vi "Loop_ACT_Drive.vi"() -> ()   [LabVIEW 2017]
uses:
  TypeDef/CLUSTER_Drive_HW_SRX_Status.ctl
  TypeDef/CLUSTER_4296_SRX_Status.ctl
  TypeDef/CLUSTER_SRX_Status Data.ctl
  TypeDef/CLUSTER_SRX_Encoder Data.ctl
  TypeDef/CLUSTER_SRX_PWM Data.ctl
  TypeDef/CLUSTER_SRX_Analog Data.ctl
  TypeDef/CLUSTER_SRX_Limit Switch Data.ctl
  TypeDef/CLUSTER_SRX_Profile Data.ctl
  TypeDef/ENUM_Drive_ACT Loop_Mode.ctl
  TypeDef/CLUSTER_Left and Right.ctl
  Globals/Global_STOP.vi
  Global_SM Write_Data Out.vi
  Global_WC_Drive_Zero_Encoders.vi
  Public/Documents/Cross The Road Electronics/Phoenix-LabVIEW/Motor Controller/Get/CTRE_Phoenix_MotorController_GetSelectedSensorData.vi
  Global_WC_Drive_Encoder_Values.vi
  Global_ACT Write_Data Out.vi
panel:
  in  "Zero Encoder":bool
  in  "D":dbl
  in  "I":dbl
  in  "P":dbl
  out "Right Data":dbl
  out "Left Data":dbl
  out "Cycle Time (S)":dbl format="%.3g"
  in  "Target Time(ms)":u32=50
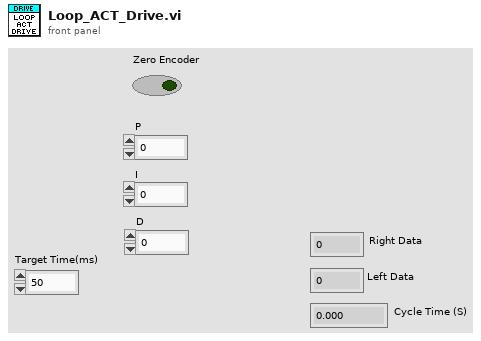
[diagram p1: front panel]
types:
  T1 = typedef "CLUSTER_Left and Right.ctl" = cluster{"Left":dbl, "Right":dbl}
  T2 = typedef "ENUM_Drive_ACT Loop_Mode.ctl" = enum16{"Stop", "Position", "VBus", "Profile"}
  T3 = typedef "CLUSTER_Drive_HW_SRX_Status.ctl" = cluster{"Rear Left":T4, "Rear Right":T4, "Front Left":T4, "Front Right":T4}
  T4 = typedef "CLUSTER_4296_SRX_Status.ctl" = cluster{"Status":T5, "Encoder":T6, "PWM ":T7, "Analog":T8, "Limit Switches":T9, "Profile":T10}
  T5 = typedef "CLUSTER_SRX_Status Data.ctl" = cluster{"Module Enabled":bool, "Current Profile Slot Select":dbl, "Brake is Enabled":bool, "Applied Throttle":dbl, "Current":dbl, "Battery Voltage":dbl, "Sticky Fault - Under Voltage":bool, "Temperature (C)":dbl, "Sticky Fault - Over Temp":bool, "CAN Error":errorcluster, "Control 5 Is Supported":bool}
  T6 = typedef "CLUSTER_SRX_Encoder Data.ctl" = cluster{"Closed Loop Error":dbl, "Sensor Position":dbl, "Sensor Velocity":dbl, "Encoder Position":dbl, "Encoder Velocity":dbl, "Encoder Index Count":dbl, "Encoder A Pin State":bool, "Encoder B Pin State":bool, "Encoder Index Pin State":bool, "Pos Div 8":bool, "Vel Div 4":bool}
  T7 = typedef "CLUSTER_SRX_PWM Data.ctl" = cluster{"Closed Loop Error":dbl, "Pulse Width Position":i32, "Pulse Width Velocity":i32, "Pulse Width Rise To Rise (us)":i32, "Pulse Width Rise To Fall (us)":i32}
  T8 = typedef "CLUSTER_SRX_Analog Data.ctl" = cluster{"Closed Loop Error":dbl, "Analog In":dbl, "Analog In Velocity":dbl}
  T9 = typedef "CLUSTER_SRX_Limit Switch Data.ctl" = cluster{"Forward Limit Switch Closed":bool, "Reverse Limit Switch Closed":bool, "Sticky Fault - Forward Limit":bool, "Sticky Fault - Reverse Limit":bool, "Sticky Fault - Forward Soft Limit":bool, "Sticky Fault - Reverse Soft Limit":bool}
  T10 = typedef "CLUSTER_SRX_Profile Data.ctl" = cluster{"Mot Prof Active Is Under Run":bool, "Mot Prof Active Has Under Run":bool, "Mot Prof Active Is Last":bool, "Mot Prof Active Velocity Only":bool, "Mot Prof Active Is Valid":bool, "Mot Prof Buffer Is Full":bool, "Mot Prof Active Profile Slot Select":i32, "Mot Prof NextID":i32, "Mot Prof Count":i32, "Mot Prof Active Velocity":dbl, "Mot Prof Active Position":dbl, "Mot Prof Output Enable":i32}
  T11 = typedef "WPI_RobotDriveDevRef.ctl" = cluster{"DevStatus":errorcluster, "Motors[]":T12[], "Square Inputs":bool, "Max Output":dbl}
  T12 = typedef "WPI_MotorControlDeviceRef.ctl" = cluster{"DeviceStatus":errorcluster, "Type":T13, "PWM":cluster{"PWM Channel":T14, "DeadBand":T15}, "CAN":cluster{"Device Number":u8, "SetOutput VI Ref":variant, "GetOutput VI Ref":variant, "Enable VI Ref":variant, "Disable VI Ref":variant, "Data":variant}, "Invert":bool, "DIO PWM":cluster{"PWM \"Enable\" Channel":T14, "DIOChannel":T16, "PWM Rate":dbl}}
  T13 = typedef "WPI_MotorControlType.ctl" = enum16{"PWM", "CAN", "DIO PWM"}
  T14 = typedef "FPGA_DIOPWMChannel.ctl" = enum8{"PWM 0", "PWM 1", "PWM 2", "PWM 3", "PWM 4", "PWM 5", "PWM 6", "PWM 7", "PWM 8", "PWM 9", "PWM MXP 0", "PWM MXP 1", "PWM MXP 2", "PWM MXP 3", "PWM MXP 4", "PWM MXP 5", "PWM MXP 6", "PWM MXP 7", "PWM MXP 8", "PWM MXP 9", "Invalid"}
  T15 = typedef "WPI_PWMDeadband.ctl" = cluster{"Name":string, "maxPositivePwm":i32, "minPositivePwm":i32, "centerPwm":i32, "maxNegativePwm":i32, "minNegativePwm":i32, "angularRange":u16}
  T16 = typedef "FPGA_DIOChannel.ctl" = enum8{"DIO 0", "DIO 1", "DIO 2", "DIO 3", "DIO 4", "DIO 5", "DIO 6", "DIO 7", "DIO 8", "DIO 9", "DIO MXP 0", "DIO MXP 1", "DIO MXP 2", "DIO MXP 3", "DIO MXP 4", "DIO MXP 5", "DIO MXP 6", "DIO MXP 7", "DIO MXP 8", "DIO MXP 9", "DIO MXP 10", "DIO MXP 11", "DIO MXP 12", "DIO MXP 13", "DIO MXP 14", "DIO MXP 15", "SPI Port CS1", "SPI Port CS2", "SPI Port CS3", "SPI Port MISO", "SPI Port MOSI", "Invalid"}
  T17 = cluster{"RobotDriveDevRef":T11, "Target Time(ms)":u32, "Current Time":timestamp, "Previous Time":timestamp, "Cycle Time (S)":dbl, "SRX_Status":T3, "Mode":T2, "VBus":T1, "Cruise RPM":dbl, "MAX Velocity\n":dbl, "Encoder Target Position":i32, "Zero Encoder":bool}
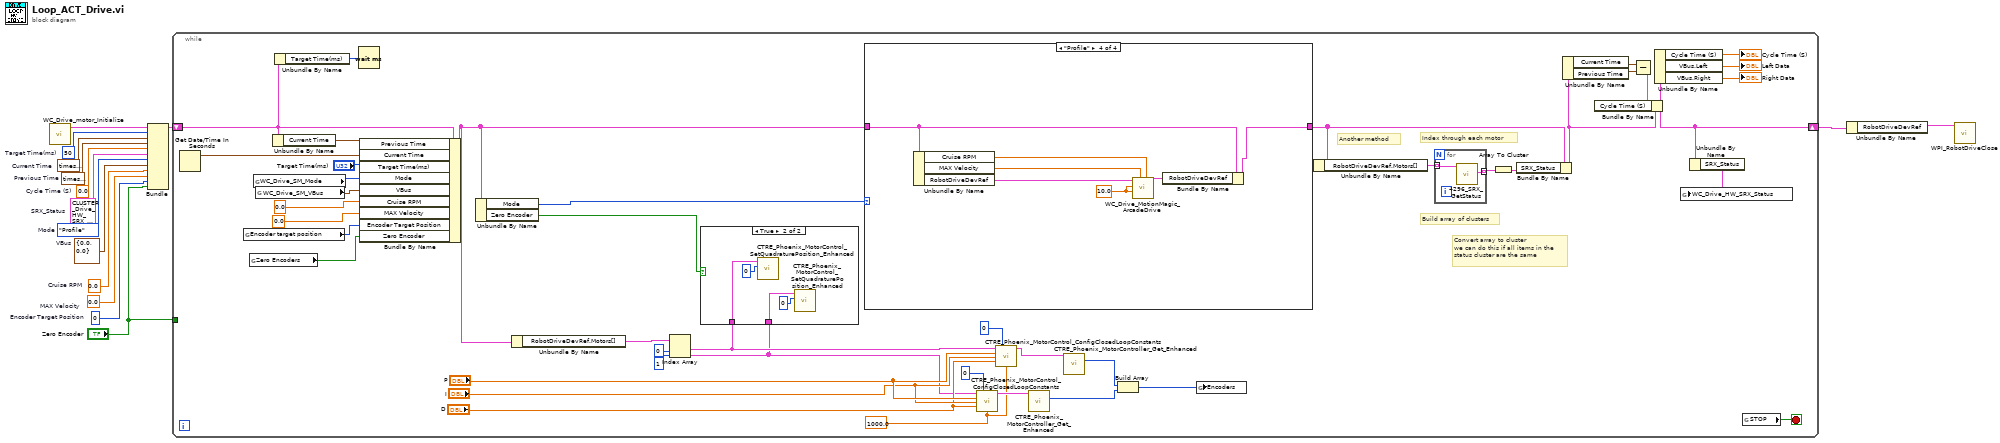
[diagram p0: block diagram]
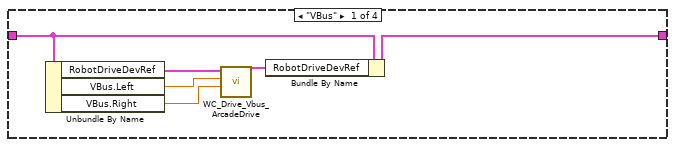
[diagram p3: hidden frame]
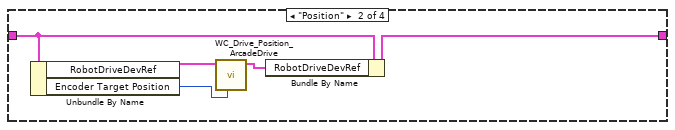
[diagram p4: hidden frame]
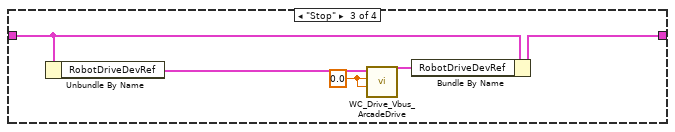
[diagram p5: hidden frame]
diagram:
  w3 = 0  # Encoder Target Position
  w4 = 0.0  # MAX Velocity
  w5 = 0.0  # Cruise RPM
  w6 = T1 {"Left"=0.0, "Right"=0.0}  # VBus
  w7 = ENUM_Drive_ACT_Loop_Mode."Profile"  # Mode
  w8 = T3 {"Rear Left"={"Status"={"Module Enabled"=FALSE, "Current Profile Slot Select"=0.0, "Brake is Enabled"=FALSE, "Applied Throttle"=0.0, "Current"=0.0, "Battery Voltage"=0.0, "Sticky Fault - Under Voltage"=FALSE, "Temperature (C)"=0.0, "Sticky Fault - Over Temp"=FALSE, "CAN Error"={"status"=FALSE, "code"=0, "source"=""}, "Control 5 Is Supported"=FALSE}, "Encoder"={"Closed Loop Error"=0.0, "Sensor Position"=0.0, "Sensor Velocity"=0.0, "Encoder Position"=0.0, "Encoder Velocity"=0.0, "Encoder Index Count"=0.0, "Encoder A Pin State"=FALSE, "Encoder B Pin State"=FALSE, "Encoder Index Pin State"=FALSE, "Pos Div 8"=FALSE, "Vel Div 4"=FALSE}, "PWM "={"Closed Loop Error"=0.0, "Pulse Width Position"=0, "Pulse Width Velocity"=0, "Pulse Width Rise To Rise (us)"=0, "Pulse Width Rise To Fall (us)"=0}, "Analog"={"Closed Loop Error"=0.0, "Analog In"=0.0, "Analog In Velocity"=0.0}, "Limit Switches"={"Forward Limit Switch Closed"=FALSE, "Reverse Limit Switch Closed"=FALSE, "Sticky Fault - Forward Limit"=FALSE, "Sticky Fault - Reverse Limit"=FALSE, "Sticky Fault - Forward Soft Limit"=FALSE, "Sticky Fault - Reverse Soft Limit"=FALSE}, "Profile"={"Mot Prof Active Is Under Run"=FALSE, "Mot Prof Active Has Under Run"=FALSE, "Mot Prof Active Is Last"=FALSE, "Mot Prof Active Velocity Only"=FALSE, "Mot Prof Active Is Valid"=FALSE, "Mot Prof Buffer Is Full"=FALSE, "Mot Prof Active Profile Slot Select"=0, "Mot Prof NextID"=0, "Mot Prof Count"=0, "Mot Prof Active Velocity"=0.0, "Mot Prof Active Position"=0.0, "Mot Prof Output Enable"=0}}, "Rear Right"={"Status"={"Module Enabled"=FALSE, "Current Profile Slot Select"=0.0, "Brake is Enabled"=FALSE, "Applied Throttle"=0.0, "Current"=0.0, "Battery Voltage"=0.0, "Sticky Fault - Under Voltage"=FALSE, "Temperature (C)"=0.0, "Sticky Fault - Over Temp"=FALSE, "CAN Error"={"status"=FALSE, "code"=0, "source"=""}, "Control 5 Is Supported"=FALSE}, "Encoder"={"Closed Loop Error"=0.0, "Sensor Position"=0.0, "Sensor Velocity"=0.0, "Encoder Position"=0.0, "Encoder Velocity"=0.0, "Encoder Index Count"=0.0, "Encoder A Pin State"=FALSE, "Encoder B Pin State"=FALSE, "Encoder Index Pin State"=FALSE, "Pos Div 8"=FALSE, "Vel Div 4"=FALSE}, "PWM "={"Closed Loop Error"=0.0, "Pulse Width Position"=0, "Pulse Width Velocity"=0, "Pulse Width Rise To Rise (us)"=0, "Pulse Width Rise To Fall (us)"=0}, "Analog"={"Closed Loop Error"=0.0, "Analog In"=0.0, "Analog In Velocity"=0.0}, "Limit Switches"={"Forward Limit Switch Closed"=FALSE, "Reverse Limit Switch Closed"=FALSE, "Sticky Fault - Forward Limit"=FALSE, "Sticky Fault - Reverse Limit"=FALSE, "Sticky Fault - Forward Soft Limit"=FALSE, "Sticky Fault - Reverse Soft Limit"=FALSE}, "Profile"={"Mot Prof Active Is Under Run"=FALSE, "Mot Prof Active Has Under Run"=FALSE, "Mot Prof Active Is Last"=FALSE, "Mot Prof Active Velocity Only"=FALSE, "Mot Prof Active Is Valid"=FALSE, "Mot Prof Buffer Is Full"=FALSE, "Mot Prof Active Profile Slot Select"=0, "Mot Prof NextID"=0, "Mot Prof Count"=0, "Mot Prof Active Velocity"=0.0, "Mot Prof Active Position"=0.0, "Mot Prof Output Enable"=0}}, "Front Left"={"Status"={"Module Enabled"=FALSE, "Current Profile Slot Select"=0.0, "Brake is Enabled"=FALSE, "Applied Throttle"=0.0, "Current"=0.0, "Battery Voltage"=0.0, "Sticky Fault - Under Voltage"=FALSE, "Temperature (C)"=0.0, "Sticky Fault - Over Temp"=FALSE, "CAN Error"={"status"=FALSE, "code"=0, "source"=""}, "Control 5 Is Supported"=FALSE}, "Encoder"={"Closed Loop Error"=0.0, "Sensor Position"=0.0, "Sensor Velocity"=0.0, "Encoder Position"=0.0, "Encoder Velocity"=0.0, "Encoder Index Count"=0.0, "Encoder A Pin State"=FALSE, "Encoder B Pin State"=FALSE, "Encoder Index Pin State"=FALSE, "Pos Div 8"=FALSE, "Vel Div 4"=FALSE}, "PWM "={"Closed Loop Error"=0.0, "Pulse Width Position"=0, "Pulse Width Velocity"=0, "Pulse Width Rise To Rise (us)"=0, "Pulse Width Rise To Fall (us)"=0}, "Analog"={"Closed Loop Error"=0.0, "Analog In"=0.0, "Analog In Velocity"=0.0}, "Limit Switches"={"Forward Limit Switch Closed"=FALSE, "Reverse Limit Switch Closed"=FALSE, "Sticky Fault - Forward Limit"=FALSE, "Sticky Fault - Reverse Limit"=FALSE, "Sticky Fault - Forward Soft Limit"=FALSE, "Sticky Fault - Reverse Soft Limit"=FALSE}, "Profile"={"Mot Prof Active Is Under Run"=FALSE, "Mot Prof Active Has Under Run"=FALSE, "Mot Prof Active Is Last"=FALSE, "Mot Prof Active Velocity Only"=FALSE, "Mot Prof Active Is Valid"=FALSE, "Mot Prof Buffer Is Full"=FALSE, "Mot Prof Active Profile Slot Select"=0, "Mot Prof NextID"=0, "Mot Prof Count"=0, "Mot Prof Active Velocity"=0.0, "Mot Prof Active Position"=0.0, "Mot Prof Output Enable"=0}}, "Front Right"={"Status"={"Module Enabled"=FALSE, "Current Profile Slot Select"=0.0, "Brake is Enabled"=FALSE, "Applied Throttle"=0.0, "Current"=0.0, "Battery Voltage"=0.0, "Sticky Fault - Under Voltage"=FALSE, "Temperature (C)"=0.0, "Sticky Fault - Over Temp"=FALSE, "CAN Error"={"status"=FALSE, "code"=0, "source"=""}, "Control 5 Is Supported"=FALSE}, "Encoder"={"Closed Loop Error"=0.0, "Sensor Position"=0.0, "Sensor Velocity"=0.0, "Encoder Position"=0.0, "Encoder Velocity"=0.0, "Encoder Index Count"=0.0, "Encoder A Pin State"=FALSE, "Encoder B Pin State"=FALSE, "Encoder Index Pin State"=FALSE, "Pos Div 8"=FALSE, "Vel Div 4"=FALSE}, "PWM "={"Closed Loop Error"=0.0, "Pulse Width Position"=0, "Pulse Width Velocity"=0, "Pulse Width Rise To Rise (us)"=0, "Pulse Width Rise To Fall (us)"=0}, "Analog"={"Closed Loop Error"=0.0, "Analog In"=0.0, "Analog In Velocity"=0.0}, "Limit Switches"={"Forward Limit Switch Closed"=FALSE, "Reverse Limit Switch Closed"=FALSE, "Sticky Fault - Forward Limit"=FALSE, "Sticky Fault - Reverse Limit"=FALSE, "Sticky Fault - Forward Soft Limit"=FALSE, "Sticky Fault - Reverse Soft Limit"=FALSE}, "Profile"={"Mot Prof Active Is Under Run"=FALSE, "Mot Prof Active Has Under Run"=FALSE, "Mot Prof Active Is Last"=FALSE, "Mot Prof Active Velocity Only"=FALSE, "Mot Prof Active Is Valid"=FALSE, "Mot Prof Buffer Is Full"=FALSE, "Mot Prof Active Profile Slot Select"=0, "Mot Prof NextID"=0, "Mot Prof Count"=0, "Mot Prof Active Velocity"=0.0, "Mot Prof Active Position"=0.0, "Mot Prof Output Enable"=0}}}  # SRX_Status
  w10 = 0.0  # Cycle Time (S)
  w15 = timestamp(0 s since 1904-01-01)  # Previous Time
  w14 = timestamp(0 s since 1904-01-01)  # Current Time
  w13 = u32 50  # Target Time(ms)
  n1 = call "WC_Drive_motor_Initialize.vi"() -> ("RobotDriveDevRef"=w2:T11)  [unwired: 11 in]
  n2 = Bundle("RobotDriveDevRef"=w2, "Target Time(ms)"=w13, "Current Time"=w14, "Previous Time"=w15, "Cycle Time (S)"=w10, "SRX_Status"=w8, "Mode"=w7, "VBus"=w6, "Cruise RPM"=w5, "MAX Velocity"=w4, "Encoder Target Position"=w3, "Zero Encoder"="Zero Encoder") -> (w12:T17)  [unwired: 1 in]
  n3 = while {
    shift-right: [w45] -> w11
    shift-left: w12 -> [w42]
    tunnel: "Zero Encoder" -> [_]
    stop <- w59 stop-if-true
    w16 = 1000.0
    # "Build array of clusters"
    # "Convert array to cluster\nwe can do this if all items in the\nstatus cluster are the same"
    # "Index through each motor"
    # "Another method"
    n4 = Get Date/Time In Seconds() -> (seconds since 1Jan1904=w58:timestamp)
    n5 = global read "Global_SM Write_Data Out.vi" "Encoder target position"() -> (w28:i32)
    n6 = global read "Global_WC_Drive_Zero_Encoders.vi" "Zero Encoders"() -> (w20:bool)
    n7 = global read "Global_SM Write_Data Out.vi" "WC_Drive_SM_Mode"() -> (w48:T2)
    n8 = global read "Global_SM Write_Data Out.vi" "WC_Drive_SM_VBus"() -> (w38:T1)
    n9 = Unbundle By Name(w42) -> ("Current Time"=w57:timestamp)
    n10 = Unbundle By Name(w42) -> ("Target Time(ms)"=w53:u32)
    n11 = Wait (ms)(milliseconds to wait=w53) -> ()  [unwired: 1 out]
    n12 = Bundle By Name(cluster=w42, "Previous Time"=w57, "Current Time"=w58, "Target Time(ms)"="Target Time(ms)", "Mode"=w48, "VBus"=w38, "Cruise RPM"=0.0, "MAX Velocity"=0.0, "Encoder Target Position"=w28, "Zero Encoder"=w20) -> (w32:T17)
    n13 = Unbundle By Name(w32) -> ("Mode"=w47:T2, "Zero Encoder"=w17:bool)
    n14 = Unbundle By Name(w32) -> ("RobotDriveDevRef.Motors[]"=w35:T12[])
    n15 = Index Array(array=w35, index #1=0 ("index"), index #2=1 ("index")) -> (element #1=w19:T12, element #2=w18:T12)
    n16 = case shown="True" w17 {
      tunnel: w19 -> [_ w63]
      tunnel: w18 -> [_ w60]
      frame False {
      }
      frame True {
        n17 = call "CTRE_Phoenix_MotorControl_SetQuadraturePosition_Enhanced.vi"("New Position"=0, "PhoenixMotorControlDevRef"=w63) -> ()  [unwired: 8 in, 2 out]
        n18 = call "CTRE_Phoenix_MotorControl_SetQuadraturePosition_Enhanced.vi"("New Position"=0, "PhoenixMotorControlDevRef"=w60) -> ()  [unwired: 8 in, 2 out]
      }
    }
    n19 = case shown="\"Profile\"" w47 {
      tunnel: w32 -> [w67 w76 w80 w84]
      tunnel: [w66 w75 w79 w85] -> w43
      frame "VBus" {
        n20 = Unbundle By Name(w67) -> ("RobotDriveDevRef"=w71:T11, "VBus.Left"=w70:dbl, "VBus.Right"=w69:dbl)
        n21 = call "WC_Drive_Vbus_ArcadeDrive.vi"("Right Value"=w69, "Left Value"=w70, "RobotDriveDevRef"=w71) -> ("RobotDriveDevRef Out"=w68:T11)  [unwired: 7 in, 1 out]
        n22 = Bundle By Name(cluster=w67, "RobotDriveDevRef"=w68) -> (w66:T17)
      }
      frame "Position" {
        n23 = Unbundle By Name(w76) -> ("RobotDriveDevRef"=w74:T11, "Encoder Target Position"=w72:i32)
        n24 = call "WC_Drive_Position_ArcadeDrive.vi"("Encoder Target Position"=w72, "RobotDriveDevRef"=w74) -> ("RobotDriveDevRef Out"=w73:T11)  [unwired: 8 in, 1 out]
        n25 = Bundle By Name(cluster=w76, "RobotDriveDevRef"=w73) -> (w75:T17)
      }
      frame "Stop" {
        w78 = 0.0 ("X axis value")
        n26 = Unbundle By Name(w80) -> ("RobotDriveDevRef"=w77:T11)
        n27 = call "WC_Drive_Vbus_ArcadeDrive.vi"("Right Value"=w78, "Left Value"=w78, "RobotDriveDevRef"=w77) -> ("RobotDriveDevRef Out"=w81:T11)  [unwired: 7 in, 1 out]
        n28 = Bundle By Name(cluster=w80, "RobotDriveDevRef"=w81) -> (w79:T17)
      }
      frame "Profile" {
        w87 = 10.0 ("X axis value")
        n29 = Unbundle By Name(w84) -> ("Cruise RPM"=w83:dbl, "MAX Velocity"=w82:dbl, "RobotDriveDevRef"=w88:T11)
        n30 = call "WC_Drive_MotionMagic_ArcadeDrive.vi"("Cruise RPM"=w83, "Max Velocity"=w82, "Right Value"=w87, "Left Value"=w87, "RobotDriveDevRef"=w88) -> ("RobotDriveDevRef Out"=w86:T11)  [unwired: 5 in, 1 out]
        n31 = Bundle By Name(cluster=w84, "RobotDriveDevRef"=w86) -> (w85:T17)
      }
    }
    n32 = call "CTRE_Phoenix_MotorControl_ConfigClosedLoopConstants.vi"("PhoenixMotorControlDevRef"=w18, "slotIdx"=0, "P"="P", "I"="I", "D"="D", "I Zone"=w16) -> ("PhoenixMotorControlDevRef"=w24:T12)  [unwired: 8 in, 1 out]
    n33 = call "CTRE_Phoenix_MotorControl_ConfigClosedLoopConstants.vi"("PhoenixMotorControlDevRef"=w19, "slotIdx"=0, "P"="P", "I"="I", "D"="D", "I Zone"=w16) -> ("PhoenixMotorControlDevRef"=w25:T12)  [unwired: 8 in, 1 out]
    n34 = call-poly "CTRE_Phoenix_MotorController_Get_Enhanced.vi"("PhoenixMotorControlDevRef"=w24) -> ("Position (Raw Sensor Units)"=w30:i32)  [unwired: 11 in, 3 out]
    n35 = call-poly "CTRE_Phoenix_MotorController_Get_Enhanced.vi"("PhoenixMotorControlDevRef"=w25) -> ("Position (Raw Sensor Units)"=w31:i32)  [unwired: 11 in, 3 out]
    n36 = Build Array(w31, w30) -> (w29:i32[])
    n37 = global write "Global_WC_Drive_Encoder_Values.vi" "Encoders"(w29) -> ()
    n38 = Unbundle By Name(w43) -> ("RobotDriveDevRef.Motors[]"=w41:T12[])
    n39 = for {
      tunnel: w41 -> [w65] mode=indexing
      tunnel: [w64] -> w40 mode=indexing
      n40 = call "4296_SRX_GetStatus.vi"("CAN Talon SRX Ref"=w65) -> ("4296 SRX Status Out"=w64:T4)  [unwired: 8 in, 2 out]
    }
    n41 = Array To Cluster(array=w40) -> (cluster=w39:cluster{"[0]":T4, "[1]":T4, "[2]":T4, "[3]":T4})
    n42 = Bundle By Name(cluster=w43, "SRX_Status"=w39) -> (w44:T17)
    n43 = Unbundle By Name(w44) -> ("Current Time"=w56:timestamp, "Previous Time"=w55:timestamp)
    n44 = Subtract(x=w56, y=w55) -> (x-y=w46:dbl)
    n45 = Bundle By Name(cluster=w44, "Cycle Time (S)"=w46) -> (w45:T17)
    n46 = Unbundle By Name(w45) -> ("Cycle Time (S)"=→"Cycle Time (S)":dbl, "VBus.Left"=→"Left Data":dbl, "VBus.Right"=→"Right Data":dbl)
    n47 = Unbundle By Name(w45) -> ("SRX_Status"=w49:T3)
    n48 = global write "Global_ACT Write_Data Out.vi" "WC_Drive_HW_SRX_Status"(w49) -> ()
    n49 = global read "Global_STOP.vi" "STOP"() -> (w59:bool)
  }
  n50 = Unbundle By Name(w11) -> ("RobotDriveDevRef"=w9:T11)
  n51 = call <vilib>:"WPI_RobotDriveClose.vi"("RobotDriveDevRef"=w9) -> ()  [unwired: 10 in, 1 out]
